vi "DMM Driver Calibration Popup.vi"(8 "error in (no error)":errorcluster, 10 "Message":string="The DMM stimulus parameters have been set, but the DMM requires normalization.\n\nPlease perform the following steps:\n\n1)  Insert a short into the the test fixture;\n2)  Press Normalize.", 11 "Header":string="Normalization of the HP 34401A DMM") -> (0 "error out":errorcluster, 3 "Button":i32)   [LabVIEW 2011]
panel:
  in  "Cancel":bool
  in  "Normalize":bool
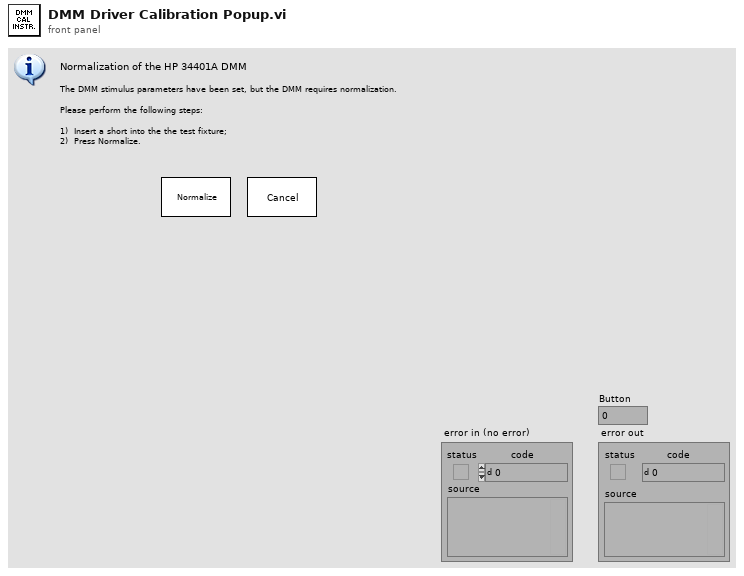
[diagram p1: front panel]
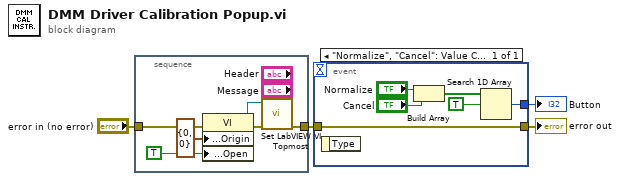
[diagram p0: block diagram]
diagram:
  n1 = stacked-sequence {
    tunnel: "error in (no error)" -> [w10]
    tunnel: [w7] -> w2
    frame #0 {
      n2 = property on="Property Node" class="VI"(error in=w10, "Front Panel Window:Origin"=cluster{"Horizontal":i16, "Vertical":i16} {"Horizontal"=0, "Vertical"=0}, "Front Panel Window:Open"=TRUE) -> (reference out=w6:refnum<vi>, error out=w8:errorcluster)  [unwired: 1 in]
      n3 = call "Set LabVIEW VI Topmost.vi"("error in (no error)"=w8, "VI Refnum (null)"=w6) -> ("error out"=w7:errorcluster)  [unwired: 7 in, 2 out]
    }
  }
  n4 = event shown="[0] \"Normalize\", \"Cancel\": Value Change" {
    selector: _ -> [_]
    dyn-events: _ -> [_]
    timeout: _ -> [_]
    tunnel: w2 -> [w16]
    tunnel: [w16] -> w4
    tunnel: [w11] -> w1
    event "Normalize", "Cancel": Value Change {
      n5 = event-data() -> ()  [unwired: 2 out]
      n6 = Build Array("Normalize", "Cancel") -> (w13:bool[])
      n7 = Search 1D Array(1D array=w13, element=TRUE) -> (index of element=w11:i32)  [unwired: 1 out]
    }
  }
  "error out" <- w4
  "Button" <- w1
